vi "Lambda_tau,T(t).vi"(8 "T-?":bool, 9 "T":dbl, 10 "tau":dbl, 11 "t":dbl) -> (3 "Lambda_[tau,T](t)":dbl format="%#_3g")   [LabVIEW 2021, in "Math.lvlib"]
uses:
  Math.lvlib
panel:
  # "set to True to compute Lambda_tau,T(T-epsilon), where epsilon -> 0"
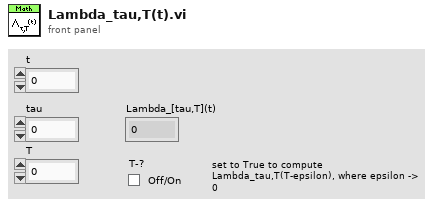
[diagram p1: front panel]
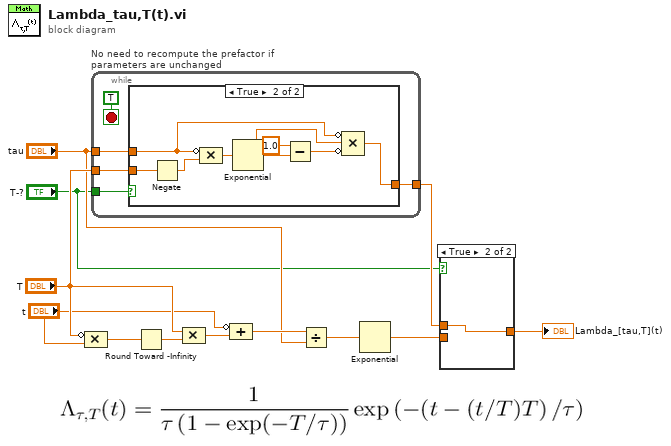
[diagram p0: block diagram]
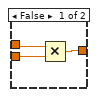
[diagram p2: hidden frame]
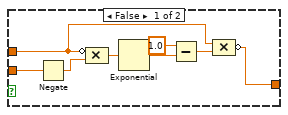
[diagram p3: hidden frame]
diagram:
  n1 = Compound Arithmetic op=MULTIPLY(invert "T", "t") -> (w12:dbl)
  n2 = while "No need to recompute the prefactor if parameters are unchanged" {
    tunnel: "T" -> [w16]
    tunnel: "tau" -> [w15]
    tunnel: "T-?" -> [w14]
    tunnel: [w13] -> w2
    stop <- TRUE stop-if-true
    n3 = case shown="True" w14 {
      tunnel: w16 -> [w25 w29]
      tunnel: w15 -> [w24 w26]
      tunnel: [w23 w27] -> w13
      frame False {
        n4 = Negate(x=w25) -> (-x=w22:dbl)
        n5 = Compound Arithmetic op=MULTIPLY(invert w24, w22) -> (w21:dbl)
        n6 = Exponential(1:w21) -> (0:w19:dbl)
        n7 = Subtract(x=1.0, y=w19) -> (x-y=w18:dbl)
        n8 = Compound Arithmetic op=MULTIPLY(w24, w18) -> (invert w23:dbl)
      }
      frame True {
        n9 = Negate(x=w29) -> (-x=w33:dbl)
        n10 = Compound Arithmetic op=MULTIPLY(invert w26, w33) -> (w32:dbl)
        n11 = Exponential(1:w32) -> (0:w28:dbl)
        n12 = Subtract(x=1.0, y=w28) -> (x-y=w30:dbl)
        n13 = Compound Arithmetic op=MULTIPLY(invert w26, w28, invert w30) -> (w27:dbl)
      }
    }
  }
  n14 = Round Toward -Infinity(1:w12) -> (0:w11:dbl)
  n15 = Compound Arithmetic op=MULTIPLY("T", w11) -> (w6:dbl)
  n16 = Compound Arithmetic op=ADD(invert "t", w6) -> (w4:dbl)
  n17 = Divide(x=w4, y="tau") -> (x/y=w10:dbl)
  n18 = Exponential(1:w10) -> (0:w9:dbl)
  n19 = case shown="True" "T-?" {
    tunnel: w9 -> [w36 _]
    tunnel: [w35 w37] -> w8
    tunnel: w2 -> [w34 w37]
    frame False {
      n20 = Multiply(x=w34, y=w36) -> (x*y=w35:dbl)
    }
    frame True {
    }
  }
  "Lambda_[tau,T](t)" <- w8
